vi "test_glo.vi"() -> ()   [LabVIEW 2012]
panel:
  in  "error-playstate":errorcluster
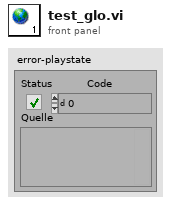
[diagram p1: front panel]
diagram:
